vi "run.create_add_label.vi"(8 "error in":errorcluster, 11 "RunCreateStaging in":refnum<class "RunCreateStaging.lvclass">) -> (0 "error out":errorcluster, 3 "RunCreateStaging out":refnum<class "RunCreateStaging.lvclass">)   [LabVIEW 2020, in "RunCreateStaging.lvclass"]
doc: "Adds a label to the run being created."
uses:
  RunCreateStaging.lvclass
  RunCreateStaging.lvclass/RunCreateStaging.ctl
  client.lvlib
panel:
  in  "label":string
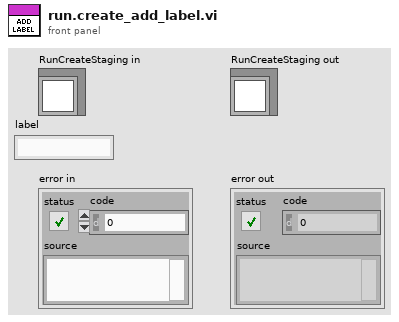
[diagram p1: front panel]
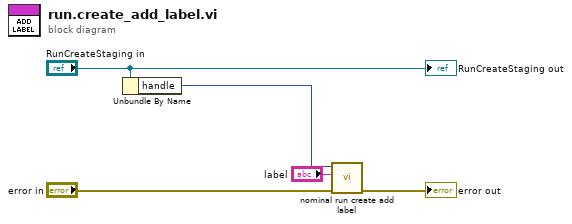
[diagram p0: block diagram]
diagram:
  n1 = Unbundle By Name("RunCreateStaging in") -> ("handle"=w3:i32)
  n2 = call "nominal run create add label.vi"("error in (no error)"="error in", "label"="label", "staging"=w3) -> ("error out"=→"error out":errorcluster)  [unwired: 7 in, 1 out]
  "RunCreateStaging out" <- "RunCreateStaging in"
